vi "checkTestComplete.vi"(8 "error in (no error)":errorcluster, 11 "TestMonitor in":refnum<class "TestMonitor.lvclass">) -> (0 "error out":errorcluster, 2 "testCompleteIsTrue":bool, 3 "TestMonitor out":refnum<class "TestMonitor.lvclass">)   [LabVIEW 2015]
uses:
  TestMonitor.lvclass
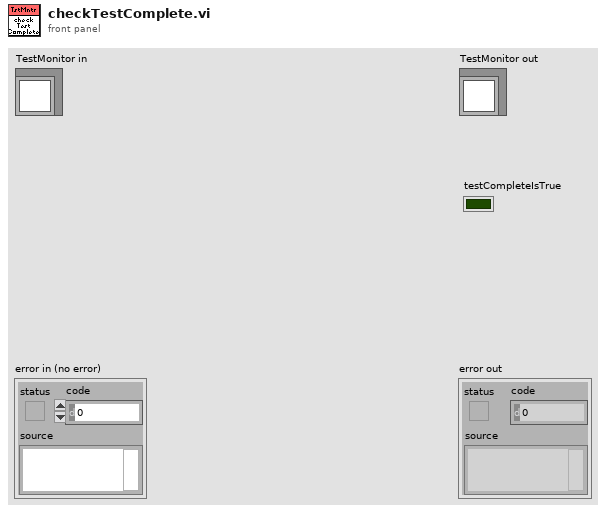
[diagram p1: front panel]
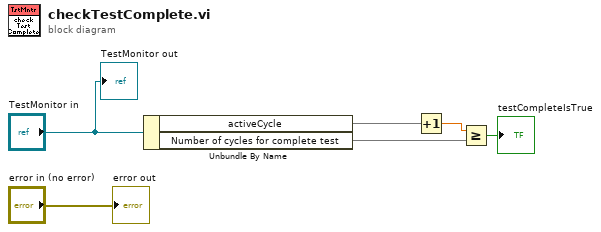
[diagram p0: block diagram]
diagram:
  n1 = Unbundle By Name("TestMonitor in") -> ("activeCycle"=w3, "Number of cycles for complete test"=w1)
  n2 = Increment(x=w3) -> (x+1=w2:dbl)
  n3 = Greater Or Equal?(x=w2, y=w1) -> (x >= y?=→"testCompleteIsTrue":bool)
  "error out" <- "error in (no error)"
  "TestMonitor out" <- "TestMonitor in"
